vi "SeCrTs-Seq DO Executer .vi"(8 "error in":errorcluster, 11 "Message Queue":refnum<queue>) -> (0 "error IO":errorcluster)   [LabVIEW 2022 SP3]
uses:
  <vilib>/Platform/TimedLoop/XDataNode/timing_clust.ctl
  <vilib>/Platform/TimedLoop/XDataNode/nitl_modes.ctl
  <vilib>/Platform/TimedLoop/XDataNode/wakeup.ctl
  d80d56e9-23fa-454b-a102-17ab65941fe7.vi
  <vilib>/platform/TimedLoop/XDataNode/XDataNode.xnode
  <vilib>/Platform/TimedLoop/XDataNode/XDNodeRunTimeDep.lvlib
panel:
  out "In Range":bool
  out "x-y":u32
  out "Numeric":i32
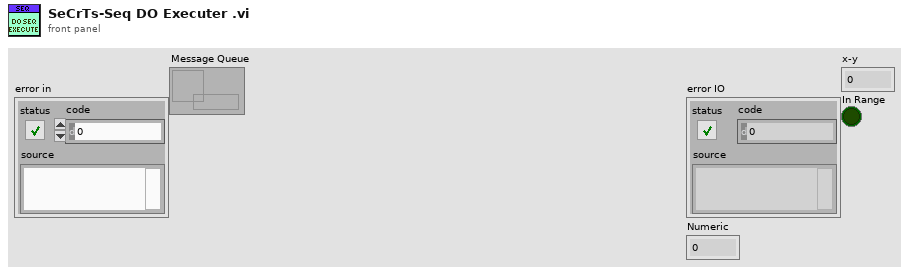
[diagram p1: front panel]
types:
  T1 = typedef "XDNodeRunTimeDep.lvlib/timing_clust.ctl" = cluster{"Expected End [f-1]":u64, "Actual End [f-1]":u64, "Finished Late? [f-1]":bool, "Expected End [i-1]":u64, "Actual End [i-1]":u64, "Finished Late? [i-1]":bool, "Expected Start [i]":u64, "Actual Start [i]":u64, "Expected Start [f]":u64, "Actual Start [f]":u64, "Source Name":string, "Structure Name":string, "Period":i64, "Deadline":i64, "Offset":i64, "Start":i64, "Priority":i32, "Timeout":i32, "Mode":T2, "Wakeup Reason":T3, "Error":errorcluster, "Source Type":string, "Secondary Source Type":string, "Global End Time":u64, "Global Start Time":u64, "Frame Duration":u64, "Iteration Duration":u64, "Assigned CPU":i32, "I/O Scan Engine Mode":u32}
  T2 = typedef "XDNodeRunTimeDep.lvlib/nitl_modes.ctl" = enum32{"No Change", "Process missed periods, maintain original phase", "Discard missed periods, maintain original phase", "Process missed periods, ignore original phase", "Discard missed periods, ignore original phase"}
  T3 = typedef "XDNodeRunTimeDep.lvlib/wakeup.ctl" = enum32{"Normal", "Aborted", "Asynchronous wakeup", "Timing source error", "Timed loop error", "Timeout"}
  T4 = enum16{"Init", "Read", "Write 'All'", "Write 'n'", "Write Safe Value", "Write Start Time", "Overwrite Pattern", "Overwrite Pattern with Start", "Append Pattern", "Start Pattern Mode", "Abort Pattern Mode", "Read 1"}
  T5 = cluster{"Manual HOLD":bool, "Automatic Hold AI":bool, "Abort":bool, "Automatic Hold DI":bool}
  T6 = cluster{"Start DAQ":bool, "Stop DAQ":bool, "RT Stop":bool, "RT Exit":bool, "Start Seq":bool}
  T7 = cluster{cluster{"Sr. No.":string, "Time CDT":string, "Component ID":string, "Data Type":string, "Condition":string, "Range/Position":string, "No of Samples for Pass":string, "Event Duration":string, "Continuous /Cumulative":string, "Expected Delay":string, "Failure case Seq":string, "Current Sequence":string}[]}[]
  T8 = cluster{"Sr. No.":string, "Time CDT":string, "Component ID":string, "Data Type":string, "Condition":string, "Range/Position":string, "No of Samples for Pass":string, "Event Duration":string, "Continuous /Cumulative":string, "Expected Delay":string, "Failure case Seq":string, "Current Sequence":string}[]
  T9 = cluster{"Sr. No.":string, "Time CDT":string, "Component ID":string, "Data Type":string, "Condition":string, "Range/Position":string, "No of Samples for Pass":string, "Event Duration":string, "Continuous /Cumulative":string, "Expected Delay":string, "Failure case Seq":string, "Current Sequence":string}
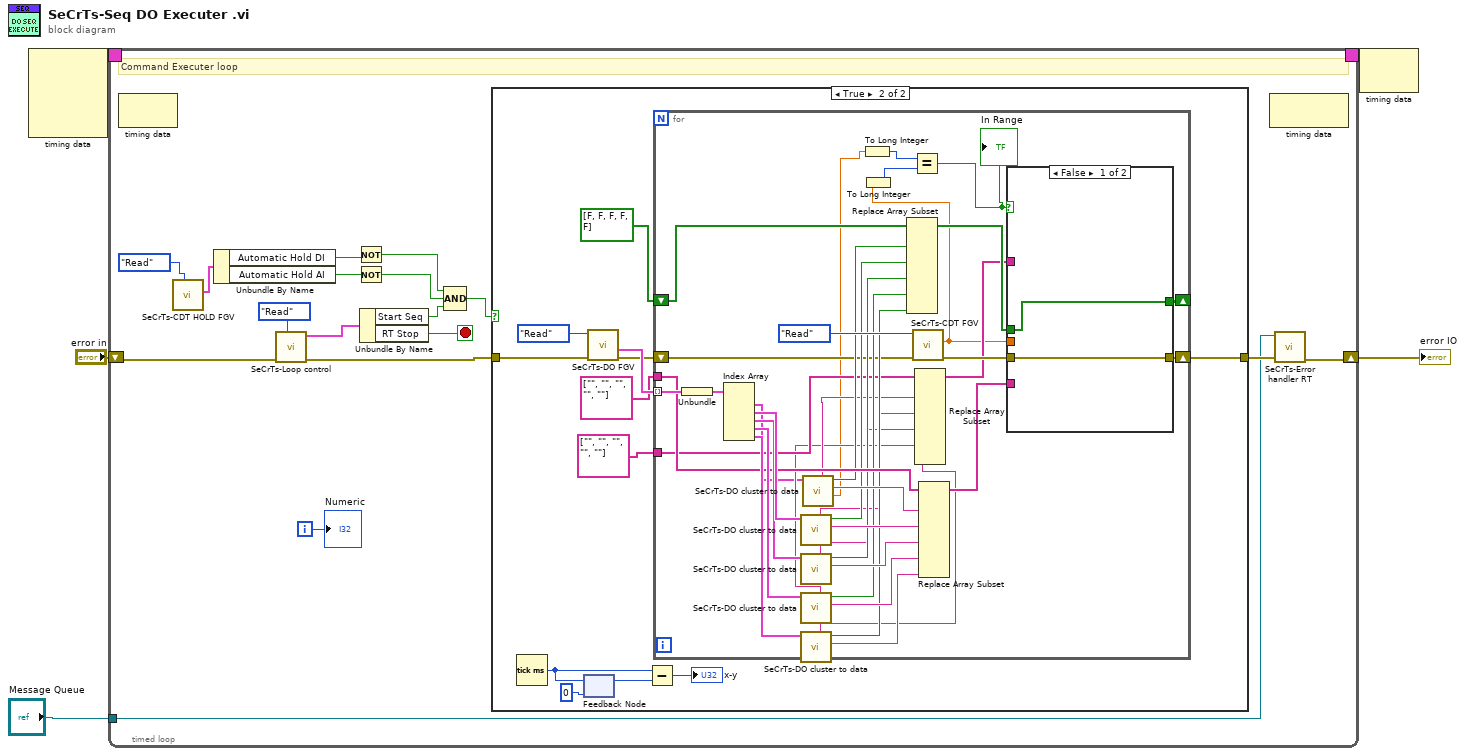
[diagram p0: block diagram]
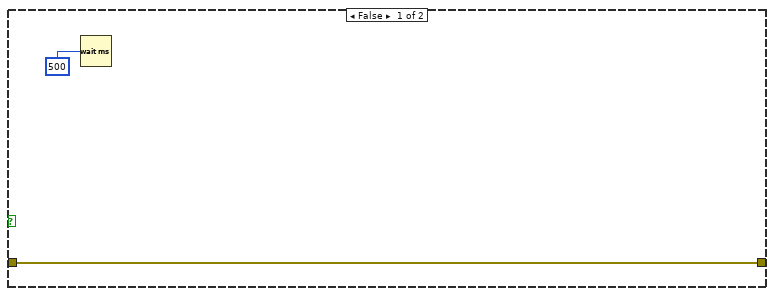
[diagram p2: hidden frame]
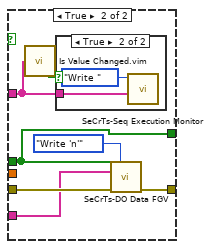
[diagram p3: hidden frame]
diagram:
  n1 = node-c288() -> (w3:T1)  [unwired: 4 in]
  n2 = timed-loop {
    shift-right: [w15] -> w4
    shift-left: "error in" -> [w20]
    timing: w3 -> [_]
    timing-out: [_] -> w2
    tunnel: "Message Queue" -> [w14]
    i -> [w21]
    stop <- w22 stop-if-true
    # "Command Executer loop"
    n3 = node-c288() -> ()  [unwired: 1 in, 1 out]
    n4 = call "SeCrTs-CDT HOLD FGV.vi"("Write/Read"=enum16{"Write", "Read"}."Read") -> ("HOLD and Abort Out"=w9:T5)  [unwired: 7 in, 1 out]
    n5 = Unbundle By Name(w9) -> ("Automatic Hold DI"=w7:bool, "Automatic Hold AI"=w8:bool)
    n6 = call "SeCrTs-Loop control.vi"("Action"=enum16{"Init", "Write", "Read"}."Read", "error in (no error)"=w20) -> ("error Out"=w19:errorcluster, "Loop Control out"=w17:T6)  [unwired: 8 in]
    n7 = Not(x=w7) -> (.not. x?=w6:bool)
    n8 = Not(x=w8) -> (.not. x?=w12:bool)
    n9 = Unbundle By Name(w17) -> ("Start Seq"=w11:bool, "RT Stop"=w22:bool)
    n10 = Compound Arithmetic op=AND(w6, w12, w11) -> (w10:bool)
    n11 = case shown="True" w10 {
      tunnel: w19 -> [w26 w36]
      tunnel: [w26 w34] -> w16
      frame False {
        n12 = Wait (ms)(milliseconds to wait=u32 500) -> ()  [unwired: 1 out]
      }
      frame True {
        n13 = Tick Count (ms)() -> (millisecond timer value=w30:u32)
        n14 = feedback #1(u32 0 ("millisecond timer value")) -> (w31:u32)
        n15 = feedback-in #1(w30) -> ()
        n16 = call "SeCrTs-DO FGV.vi"("error in"=w36, "Enum"=enum16{"Read", "Write "}."Read") -> ("error out"=w35:errorcluster, "DO Seq  OUT"=w37:T7)  [unwired: 8 in]
        n17 = Subtract(x=w30, y=w31) -> (x-y=→"x-y":u32)
        n18 = for {
          tunnel: w37 -> [w76] mode=indexing
          tunnel: string[] ["", "", "", "", ""] ("appended array") -> [w68]
          shift-right: [w69] -> w34
          shift-left: w35 -> [w54]
          tunnel: string[] ["", "", "", "", ""] ("appended array") -> [w52]
          shift-right: [w44] -> _
          shift-left: bool[] [FALSE, FALSE, FALSE, FALSE, FALSE] ("appended array") -> [w61]
          n19 = Unbundle(w76) -> (w75:T8)
          n20 = Index Array(array=w75) -> (element #1=w45:T9, element #2=w74:T9, element #3=w73:T9, element #4=w72:T9, element #5=w71:T9)  [unwired: 5 in]
          n21 = call "SeCrTs-DO cluster to data.vi"("output cluster"=w74) -> ("Component ID"=w66:string, "Boolean"=w60:bool, "Sequence"=w50:string)  [unwired: 7 in, 1 out]
          n22 = call "SeCrTs-DO cluster to data.vi"("output cluster"=w73) -> ("Component ID"=w65:string, "Boolean"=w59:bool, "Sequence"=w49:string)  [unwired: 7 in, 1 out]
          n23 = call "SeCrTs-DO cluster to data.vi"("output cluster"=w72) -> ("Component ID"=w64:string, "Boolean"=w58:bool, "Sequence"=w47:string)  [unwired: 7 in, 1 out]
          n24 = call "SeCrTs-DO cluster to data.vi"("output cluster"=w71) -> ("Component ID"=w63:string, "Boolean"=w57:bool, "Sequence"=w46:string)  [unwired: 7 in, 1 out]
          n25 = call "SeCrTs-DO cluster to data.vi"("output cluster"=w45) -> ("Numeric"=w40:dbl, "Component ID"=w67:string, "Boolean"=w62:bool, "Sequence"=w51:string)  [unwired: 7 in]
          n26 = To Long Integer(number=w40) -> (32bit integer=w39:i32)
          n27 = Replace Array Subset(array=w61, new element #1=w62, new element #2=w60, new element #3=w59, new element #4=w58, new element #5=w57) -> (w56:bool[])  [unwired: 5 in]
          n28 = call "SeCrTs-CDT FGV.vi"("error in (no error)"=w54, "Write/Read"=enum16{"Write", "Read"}."Read") -> ("error Out"=w53:errorcluster, "CDT Out"=w43:dbl)  [unwired: 8 in]
          n29 = To Long Integer(number=w43) -> (32bit integer=w41:i32)
          n30 = Equal?(x=w39, y=w41) -> (x = y?=w42:bool)
          "In Range" <- w42
          n31 = Replace Array Subset(array=w52, new element #1=w51, new element #2=w50, new element #3=w49, new element #4=w47, new element #5=w46) -> (w48:string[])  [unwired: 5 in]
          n32 = Replace Array Subset(array=w68, new element #1=w67, new element #2=w66, new element #3=w65, new element #4=w64, new element #5=w63) -> (w55:string[])  [unwired: 5 in]
          n33 = case shown="False" w42 {
            tunnel: w53 -> [w78 w85]
            tunnel: [w78 w84] -> w69
            tunnel: w43 -> [_ _]
            tunnel: w56 -> [w77 w79]
            tunnel: w55 -> [_ w83]
            tunnel: w48 -> [_ w81]
            tunnel: [w77 w79] -> w44
            frame False {
            }
            frame True {
              n34 = call "Is Value Changed.vim"("value"=w81) -> ("changed or first call?"=w80:bool)
              n35 = case shown="True" w80 {
                tunnel: w81 -> [_ w86]
                frame False {
                }
                frame True {
                  n36 = call "SeCrTs-Seq Execution Monitor.vi"("Seq Monitor"=w86, "Enum"=enum16{"Read", "Write "}."Write ") -> ()  [unwired: 8 in, 2 out]
                }
              }
              n37 = call "SeCrTs-DO Data FGV.vi"("DO Values In"=w79, "Option"=T4."Write 'n'", "DO Channel Names"=w83, "error in (no error)"=w85) -> ("error out"=w84:errorcluster)  [unwired: 5 in, 6 out]
            }
          }
        }
      }
    }
    n38 = node-c288() -> ()  [unwired: 1 in, 1 out]
    n39 = call "SeCrTs-Error handler RT.vi"("error in"=w16, "Message Queue"=w14) -> ("error out"=w15:errorcluster)  [unwired: 8 in, 1 out]
    "Numeric" <- w21
  }
  "error IO" <- w4
  n40 = node-c288(w2) -> ()  [unwired: 1 out]
